vi "IMAQdx Acquisition Template (Host)fortest.vi"() -> ()   [LabVIEW 2016]
uses:
  <vilib>/userdefined/High Color/IMAQdx.ctl
  <vilib>/FPGAPlugInAG/roboRIO/niLvFpga_Open_roboRIO.vi
  <vilib>/rvi/interface/common/dynamic/niFpgaDynamicAddResources.vi
  <vilib>/FPGAPlugInAG/Dynamic/niLvFpga_Download_Dynamic.vi
  <vilib>/FPGAPlugInAG/Dynamic/niLvFpga_Run_Dynamic.vi
  <vilib>/FPGAPlugInAG/Dynamic/niLvFpga_Close_Dynamic.vi
  <vilib>/Utility/error.llb/Error Cluster From Error Code.vi
  <vilib>/rvi/errors/niLvFpgaAdjustHostInterfaceError.vi
  <vilib>/rvi/interface/nirviOpenFPGA/nirviOpenFPGA.xnode
  FPGA Bitfiles/ImageProcessingw_FPGATarget_ImageProcessingw_Z23Lc7CsNwk.lvbitx
  <vilib>/rvi/interface/nirviMethod/nirviMethod.xnode
  <vilib>/rvi/interface/nirviCloseFPGA/nirviCloseFPGA.xnode
  <vilib>/rvi/interface/nirviReadWriteControl/nirviReadWriteControl.xnode
  <vilib>/vision/driver/NI_Vision_Acquisition_Software.lvlib
  <resource>/objmgr/imaqdx.rc
  <vilib>/rvi/interface/Simulation/niFpgaSimulationCallBeginRW.vi
  NiFpgaLv.dll
panel:
  out "Error Out 2":errorcluster
  in  "Stop":bool
  in  "Camera":T1="cam0"
  # "Overview: Demonstrates how to acquire an image from a camera using the IMAQdx API, transfer the image to a FPGA target for processing, and retrieve the processed image for display or further processing on the host.\nRequirements:\n- LabVIEW FPGA\n- Vision Acquisition Software\n- Vision Development Module\nInstructions:\n1. Select a Camera\n2. Run the VI."
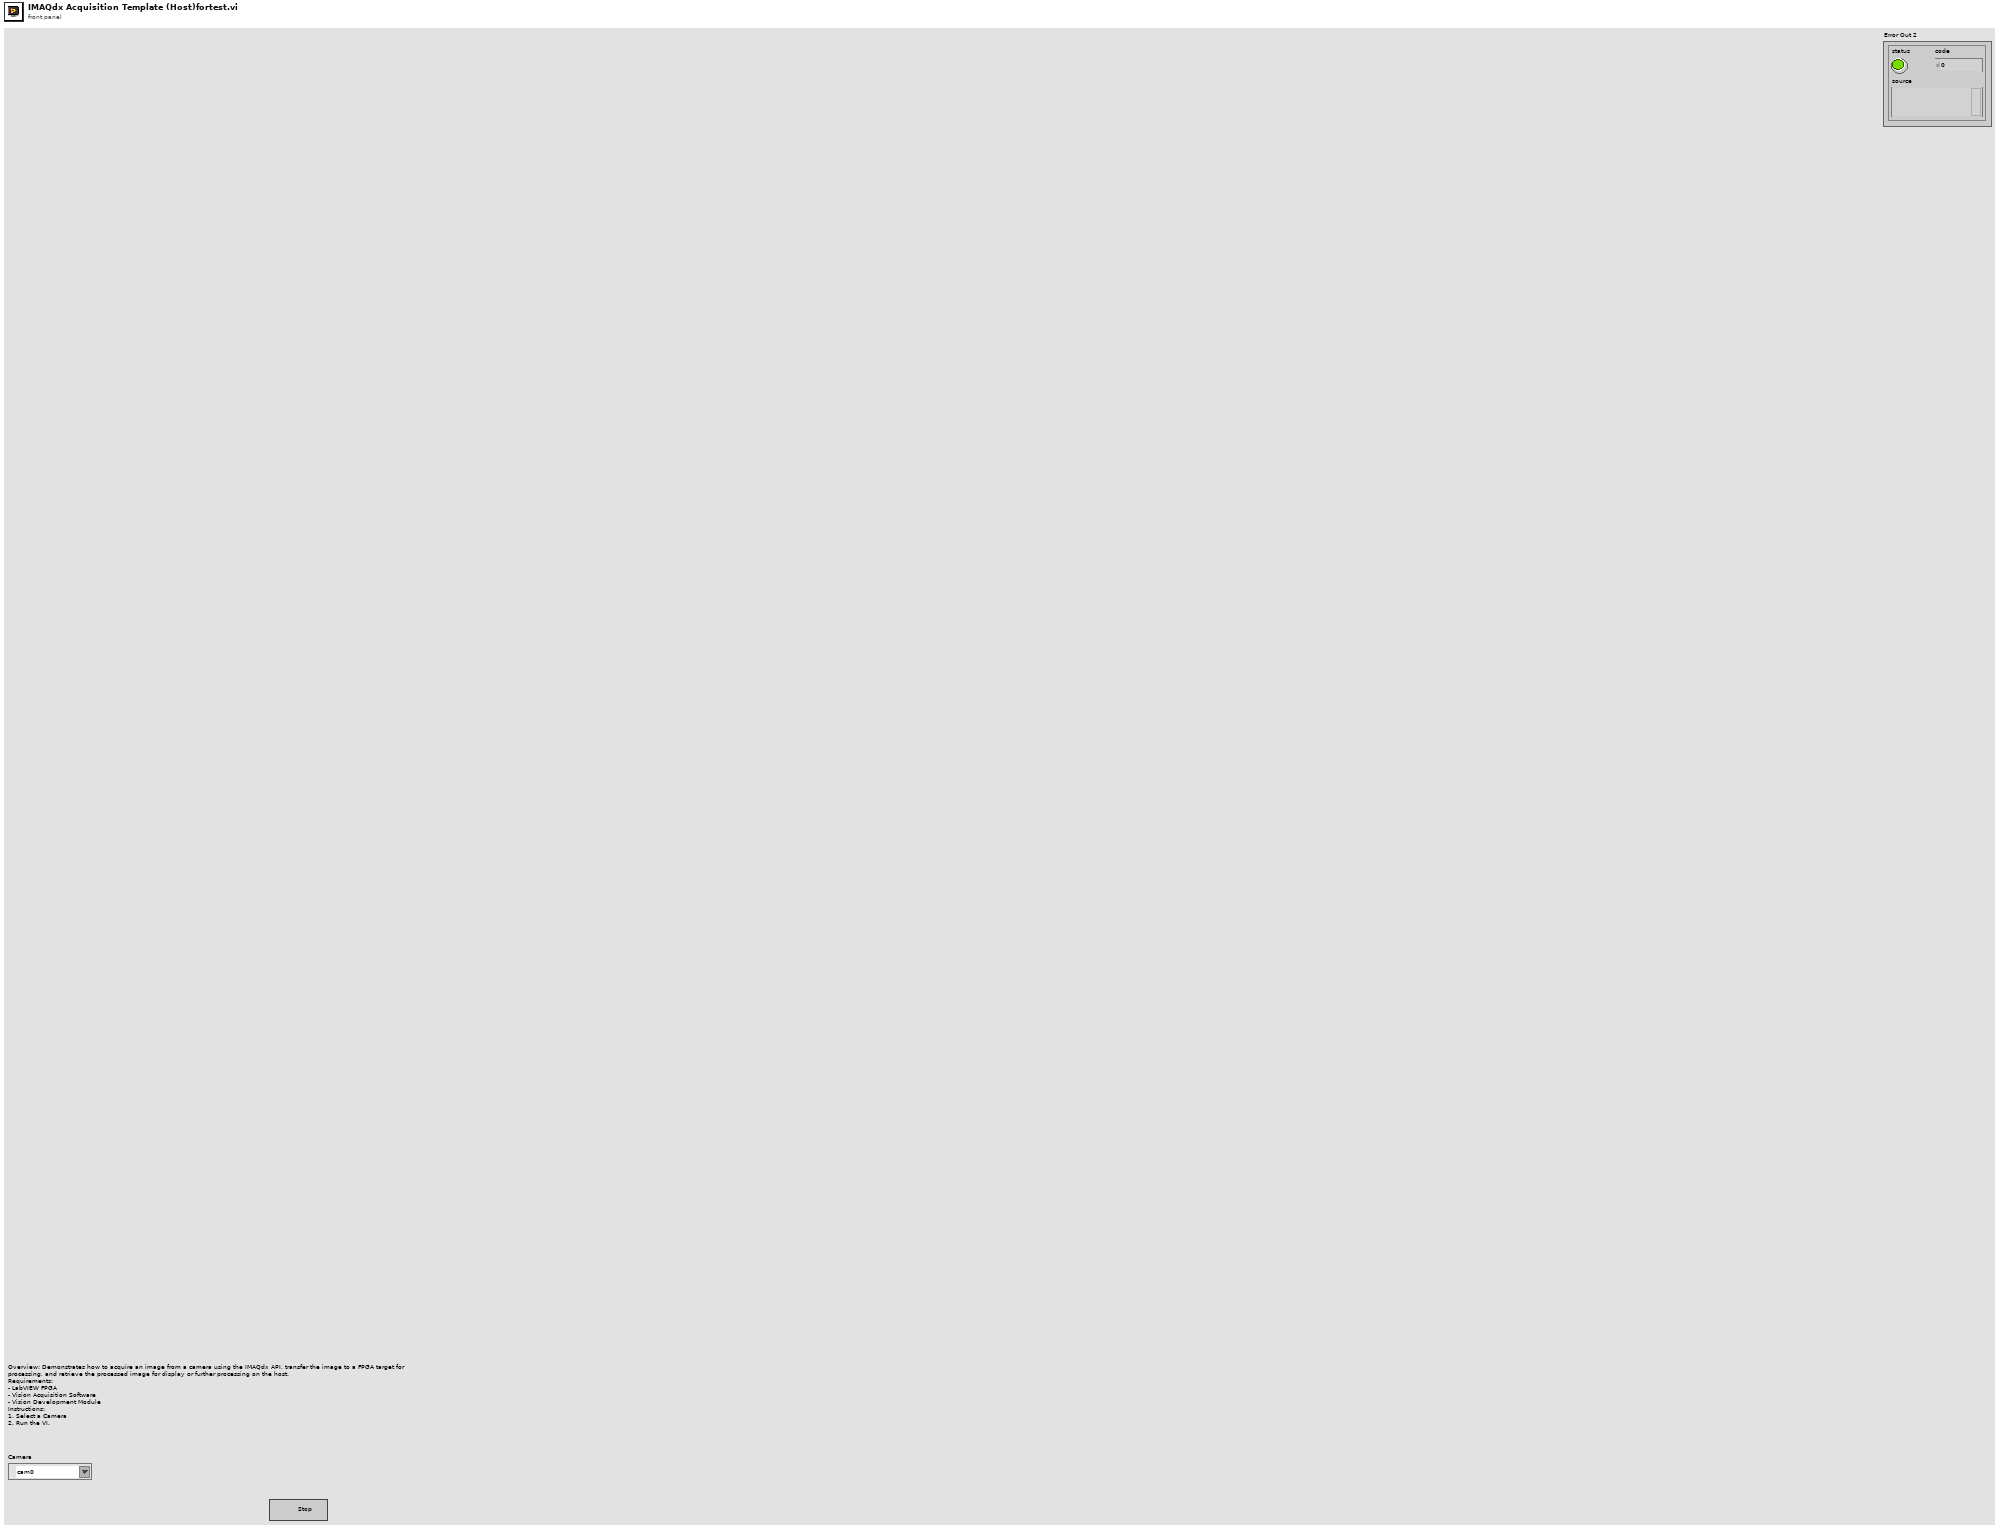
[diagram p1: front panel]
types:
  T1 = typedef "IMAQdx.ctl" = refnum<k21>
  T2 = typedef "Image Type" = u32
  T3 = typedef "IMAQ Image.ctl" = refnum<image>
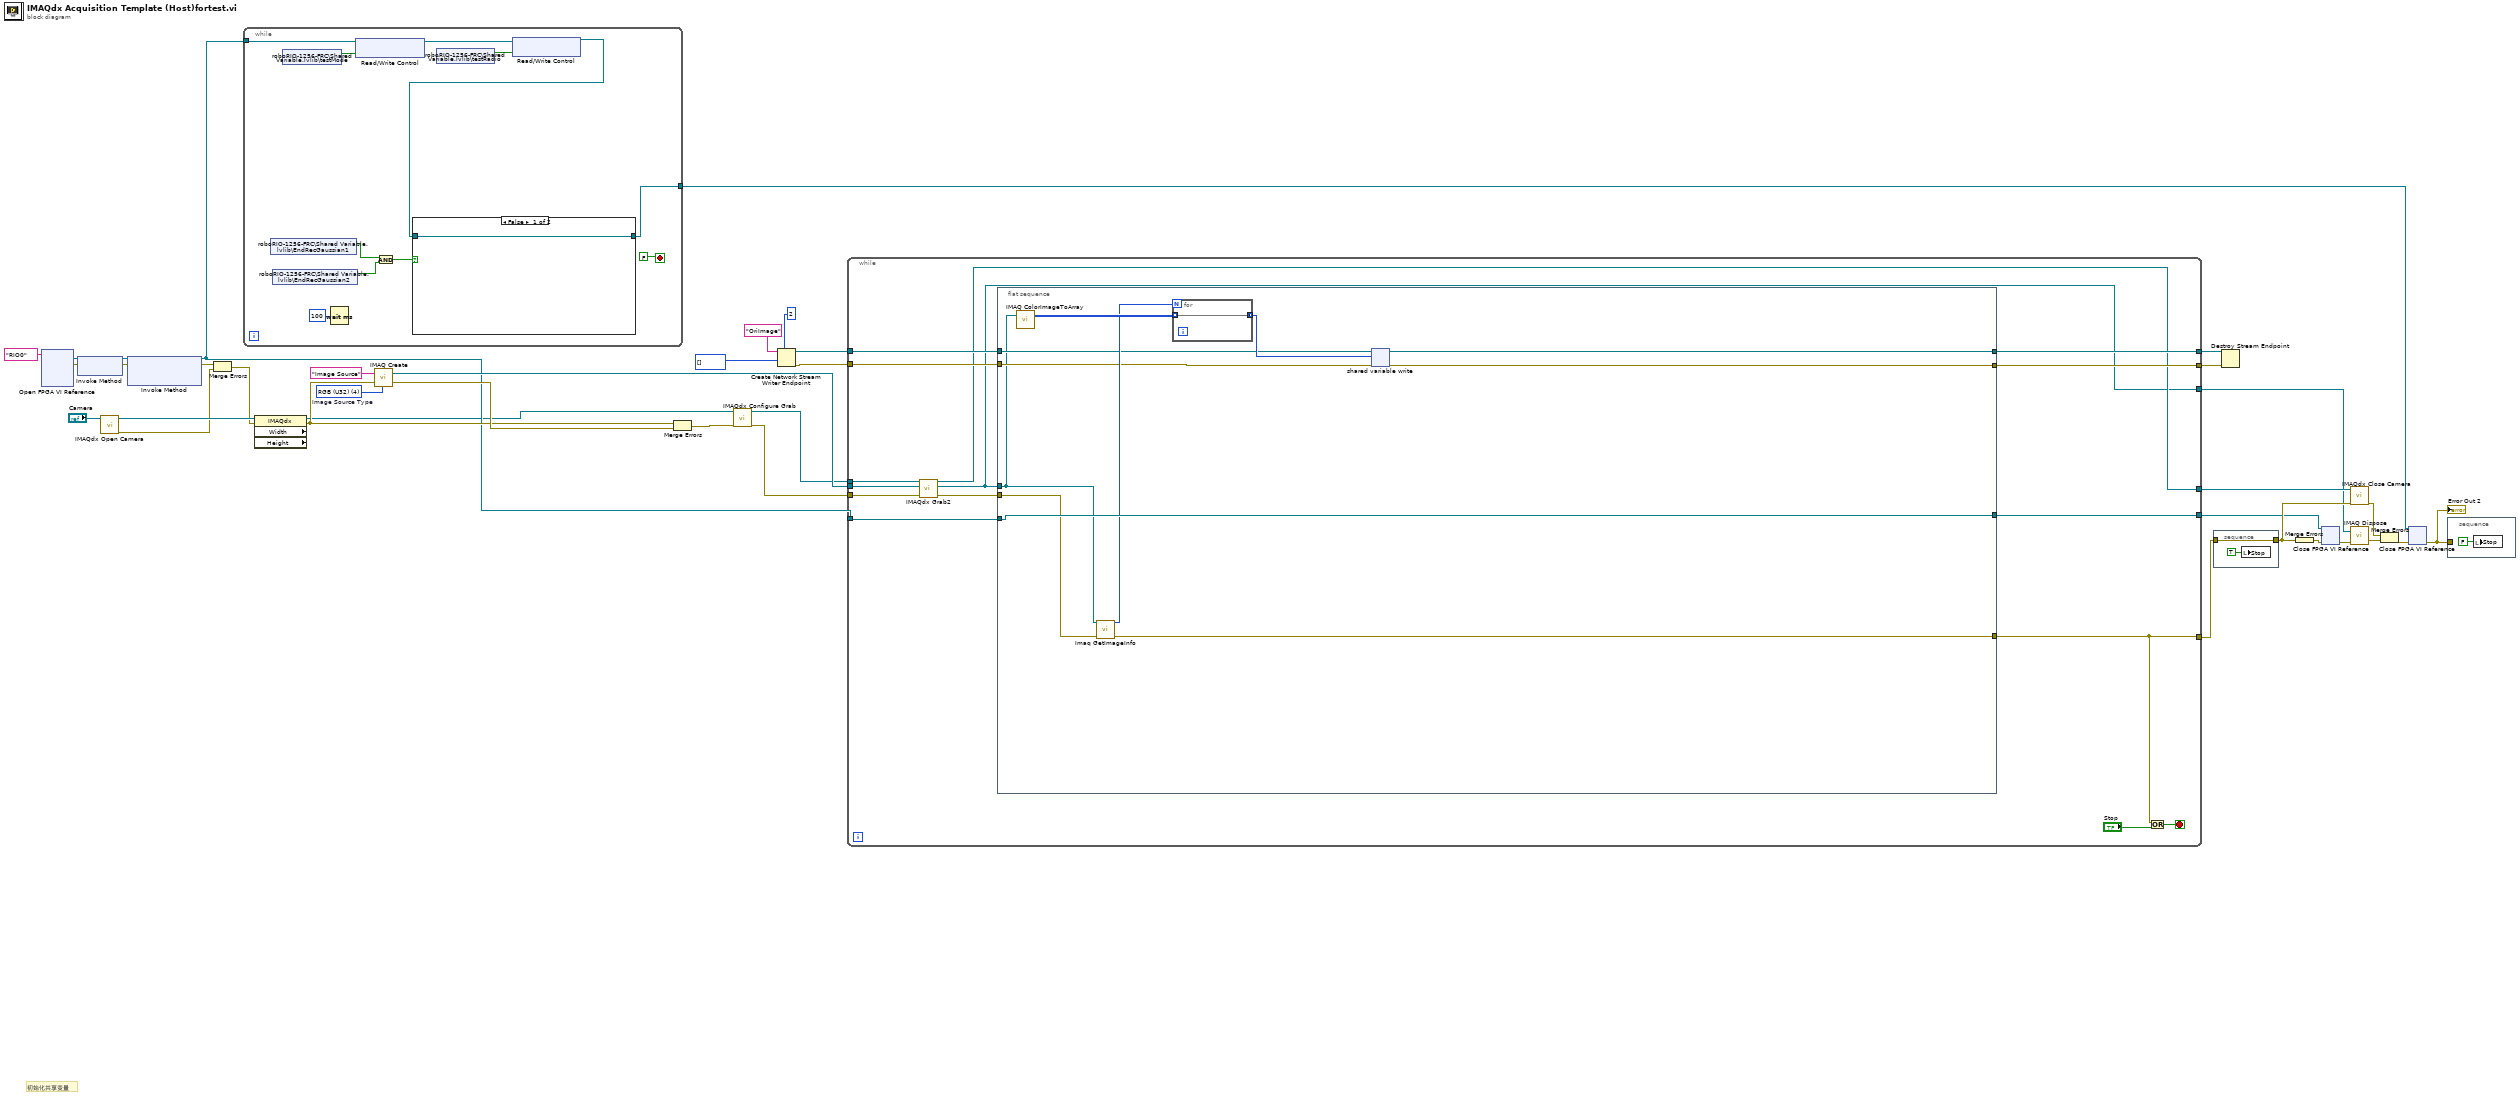
[diagram p0: block diagram]
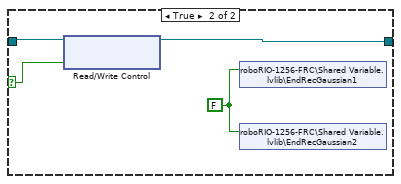
[diagram p2: hidden frame]
diagram:
  w28 = T2 4 items=["Grayscale (U8)", "Grayscale (I16)", "Grayscale (SGL)", "Complex (CSG)", "RGB (U32)", "HSL (U32)", "RGB (U64)", "Grayscale (U16)"]  # Image Source Type
  # "初始化共享变量"
  n1 = xnode "Open FPGA VI Reference"("resource name"=tag "RIO0") -> ("FPGA VI Reference Out"=w35:refnum<k20>, "error out"=w36:errorcluster)  [unwired: 1 in]
  n2 = xnode "Invoke Method"("FPGA VI Reference In"=w35, "error in"=w36) -> ("FPGA VI Reference Out"=w38:refnum<k20>, "error out"=w37:errorcluster)
  n3 = call <vilib>:"IMAQdx Open Camera.vi"("Session In"="Camera") -> ("error out"=w30:errorcluster, "Session Out"=w31:T1)  [unwired: 9 in]
  n4 = xnode "Invoke Method"("FPGA VI Reference In"=w38, "error in"=w37) -> ("FPGA VI Reference Out"=w5:refnum<k20>, "error out"=w32:errorcluster)  [unwired: 1 in]
  n5 = Merge Errors(w32, w30) -> (w29:errorcluster)
  n6 = while {
    tunnel: w5 -> [w45]
    tunnel: [w40] -> w7
    stop <- FALSE stop-if-true
    n7 = shared-variable "roboRIO-1256-FRC\\Shared Variable.lvlib\\EndRecGaussian1"() -> (w49:bool)  [unwired: 1 in, 1 out]
    n8 = shared-variable "roboRIO-1256-FRC\\Shared Variable.lvlib\\EndRecGaussian2"() -> (w48:bool)  [unwired: 1 in, 1 out]
    n9 = shared-variable "roboRIO-1256-FRC\\Shared Variable.lvlib\\testMode"() -> (w44:bool)  [unwired: 1 in, 1 out]
    n10 = Wait (ms)(milliseconds to wait=u32 100) -> ()  [unwired: 1 out]
    n11 = xnode "Read/Write Control"("FPGA VI Reference In"=w45, "Mode LED Status"=w44) -> ("FPGA VI Reference Out"=w43:refnum<k20>)  [unwired: 1 in, 1 out]
    n12 = And(x=w49, y=w48) -> (x .and. y?=w47:bool)
    n13 = shared-variable "roboRIO-1256-FRC\\Shared Variable.lvlib\\testRadio"() -> (w42:bool)  [unwired: 1 in, 1 out]
    n14 = xnode "Read/Write Control"("FPGA VI Reference In"=w43, "Radio LED Status"=w42) -> ("FPGA VI Reference Out"=w41:refnum<k20>)  [unwired: 1 in, 1 out]
    n15 = case shown="False" w47 {
      selector: w47 -> [_ w53]
      tunnel: w41 -> [w51 w55]
      tunnel: [w51 w52] -> w40
      frame False {
      }
      frame True {
        w54 = FALSE
        n16 = xnode "Read/Write Control"("FPGA VI Reference In"=w55, "StartOfImage"=w53) -> ("FPGA VI Reference Out"=w52:refnum<k20>)  [unwired: 1 in, 1 out]
        n17 = shared-variable "roboRIO-1256-FRC\\Shared Variable.lvlib\\EndRecGaussian1"(w54) -> ()  [unwired: 1 in, 1 out]
        n18 = shared-variable "roboRIO-1256-FRC\\Shared Variable.lvlib\\EndRecGaussian2"(w54) -> ()  [unwired: 1 in, 1 out]
      }
    }
  }
  n19 = property class="IMAQdx" props=["Width", "Height"](reference=w31, error in=w29) -> (reference out=w4:T1, error out=w26:errorcluster)  [unwired: 2 out]
  n20 = call "IMAQ Create"("Image Name"="Image Source", "Image Type"=w28, "error in (no error)"=w26) -> ("New Image"=w6:T3, "error out"=w27:errorcluster)  [unwired: 2 in]
  n21 = Merge Errors(w26, w27) -> (w3:errorcluster)
  n22 = call <vilib>:"IMAQdx Configure Grab.vi"("error in"=w3, "Session In"=w4) -> ("error out"=w1:errorcluster, "Session Out"=w2:T1)  [unwired: 8 in]
  n23 = Create Network Stream Writer Endpoint(7:2 ("writer buffer size"), 9:i32[] [], 11:"OriImage" ("writer name")) -> (0:w19:errorcluster, 3:w20:refnum<k21>)  [unwired: 4 in]
  n24 = while {
    tunnel: [w68] -> w25
    tunnel: [w67] -> w24
    tunnel: w20 -> [w66]
    tunnel: w19 -> [w65]
    tunnel: [w58] -> w11
    tunnel: w2 -> [w61]
    tunnel: w6 -> [w60]
    tunnel: w1 -> [w59]
    tunnel: w5 -> [w62]
    tunnel: [w64] -> w9
    tunnel: [w63] -> w10
    tunnel: [w57] -> w8
    stop <- w69 stop-if-true
    n25 = call <vilib>:"IMAQdx Grab2.vi"("error in"=w59, "Image In"=w60, "Session In"=w61) -> ("error out"=w56:errorcluster, "Image Out"=w57:T3, "Session Out"=w58:T1)  [unwired: 5 in, 1 out]
    n26 = flat-sequence {
      tunnel: [w81] -> w64
      tunnel: [w76] -> w68
      tunnel: [w75] -> w67
      tunnel: [w80] -> w63
      tunnel: w62 -> [w80]
      tunnel: w66 -> [w74]
      tunnel: w65 -> [w73]
      tunnel: w56 -> [w72]
      tunnel: w57 -> [w71]
      frame #0 {
        n27 = call "IMAQ ColorImageToArray"("Image"=w71) -> ("Image Pixels (U32)"=w79:u32[][])  [unwired: 3 in, 2 out]
        n28 = call "Imaq GetImageInfo"("error in (no error)"=w72, "Image"=w71) -> ("error out"=w81:errorcluster, "X Resolution"=w78:i32)  [unwired: 2 in, 6 out]
        n29 = for {
          N: w78 -> [_]
          tunnel: w79 -> [w82] mode=indexing
          tunnel: [w82] -> w77 mode=concatenating
        }
        n30 = shared-variable-write(w74, w73, w77) -> (w76:refnum<k21>, w75:errorcluster)  [unwired: 1 in, 1 out]
      }
    }
    n31 = Or(x=w64, y="Stop") -> (x .or. y?=w69:bool)
  }
  n32 = stacked-sequence {
    tunnel: w9 -> [w83]
    tunnel: [w83] -> w12
    frame #0 {
      n33 = local write "Stop"(TRUE ("Stop")) -> ()
    }
  }
  n34 = Destroy Stream Endpoint(8:w24, 11:w25) -> ()  [unwired: 1 out]
  n35 = Merge Errors(w12) -> (w13:errorcluster)
  n36 = xnode "Close FPGA VI Reference"("FPGA VI Reference In"=w10, "error in"=w13) -> ("error out"=w18:errorcluster)
  n37 = call <vilib>:"IMAQdx Close Camera.vi"("error in"=w12, "Session In"=w11) -> ("error out"=w16:errorcluster)  [unwired: 9 in]
  n38 = call "IMAQ Dispose"("Image"=w8, "error in (no error)"=w18) -> ("error out"=w17:errorcluster)  [unwired: 4 in]
  n39 = Merge Errors(w16, w17) -> (w15:errorcluster)
  n40 = xnode "Close FPGA VI Reference"("FPGA VI Reference In"=w7, "error in"=w15) -> ("error out"=w14:errorcluster)
  "Error Out 2" <- w14
  n41 = stacked-sequence {
    tunnel: w14 -> [_]
    frame #0 {
      n42 = local write "Stop"(FALSE ("Stop")) -> ()
    }
  }
